vi "FTW-Endpoint-Pipe-Construct.vi"(0 "FTW Endpoint":refnum<class "FTW-Endpoint.lvclass">, 5 "Address":string, 7 "Requested Identity":string, 9 "Size (-1)":i32=-1, 11 "error in":errorcluster) -> (4 "FTW Endpoint out":refnum<class "FTW-Endpoint.lvclass">, 8 "Actual Identity":string, 15 "error out":errorcluster)   [LabVIEW 2013, in "FTW-Endpoint.lvclass"]
uses:
  FTW-Endpoint.lvclass
  FTW-Endpoint.lvclass/FTW-Endpoint.ctl
  Message/FTW-Message.ctl
panel:
  # "Inputs"
  # "Outputs"
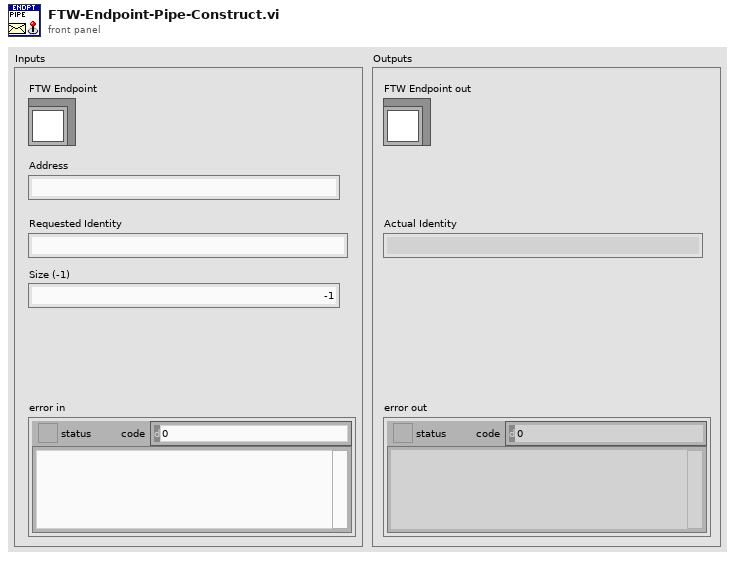
[diagram p1: front panel]
types:
  T1 = typedef "FTW-Message.ctl" = cluster{"Header":string, "Body":string, "Metadata":string}
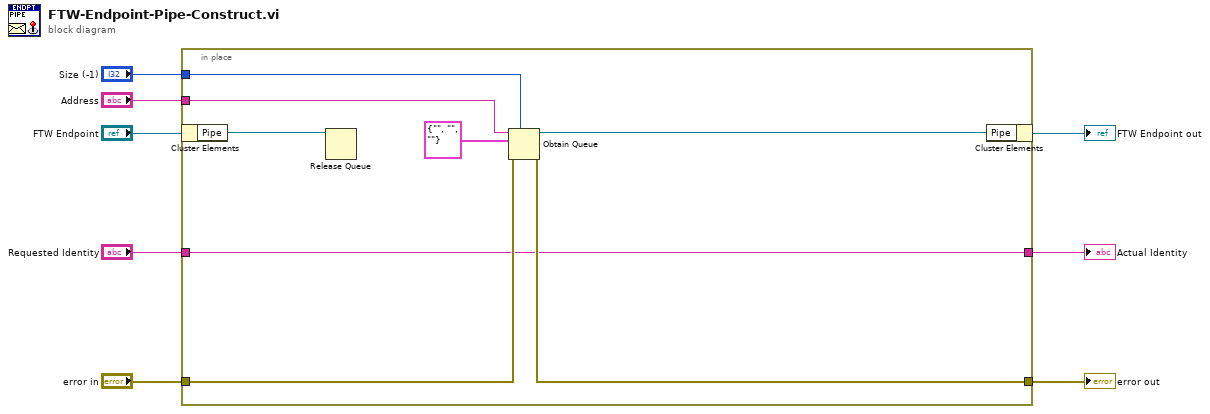
[diagram p0: block diagram]
diagram:
  n1 = in-place {
    in-place-border: "Requested Identity" -> [w12]
    in-place-border: "error in" -> [w15]
    in-place-border: [w13] -> w8
    in-place-border: [w12] -> w3
    in-place-border: "Address" -> [w11]
    in-place-border: "Size (-1)" -> [w10]
    n2 = in-place-cluster #1("FTW Endpoint") -> ("Pipe"=w16:refnum<queue>)
    n3 = Release Queue(queue=w16) -> ()  [unwired: 2 in, 3 out]
    n4 = Obtain Queue(max queue size (-1, unlimited)=w10, name (unnamed)=w11, element data type=T1 {"Header"="", "Body"="", "Metadata"=""} ("Message"), error in (no error)=w15) -> (queue out=w14:refnum<queue>, error out=w13:errorcluster)  [unwired: 1 in, 1 out]
    n5 = in-place-cluster #1("Pipe"=w14) -> (→"FTW Endpoint out":refnum<class "FTW-Endpoint.lvclass">)
  }
  "error out" <- w8
  "Actual Identity" <- w3
